vi "ParseCreators.vi"(11 "Raw HTML":string) -> (3 "Creators":T1[](array[typedef]))   [LabVIEW 2022 SP3]
uses:
  TypeDefs/Creator.ctl
  <vilib>/Utility/error.llb/Trim Whitespace One-Sided.vi
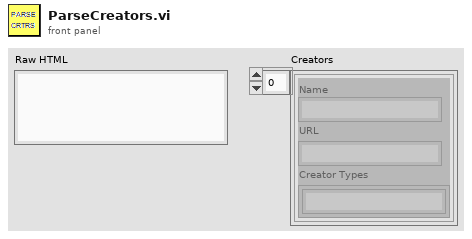
[diagram p1: front panel]
types:
  T1 = typedef "Creator.ctl" = cluster{"Name":string, "URL":string, "Creator Types":string[]}
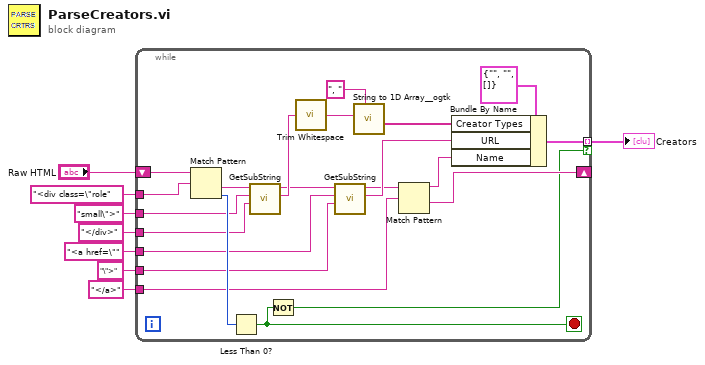
[diagram p0: block diagram]
diagram:
  n1 = while {
    shift-right: [w16] -> _
    shift-left: "Raw HTML" -> [w30]
    tunnel: "<div class=\"role" -> [w29]
    tunnel: "</div>" -> [w26]
    tunnel: "small\">" -> [w25]
    tunnel: "<a href=\"" -> [w22]
    tunnel: "\">" -> [w21]
    tunnel: "</a>" -> [w18]
    tunnel: [w15] -> w1 mode=indexing if=w13
    stop <- w14 stop-if-true
    n2 = Match Pattern(string=w30, regular expression=w29) -> (after substring=w27:string, offset past match=w28:i32)  [unwired: 1 in, 2 out]
    n3 = Less Than 0?(x=w28) -> (x < 0?=w14:bool)
    n4 = call "GetSubString.vi"("End Search"=w26, "Start Search"=w25, "String In"=w27) -> ("Match"=w24:string, "Following String Out"=w23:string)  [unwired: 6 in, 1 out]
    n5 = Not(x=w14) -> (.not. x?=w13:bool)
    n6 = call <vilib>:"Trim Whitespace.vi"("string"=w24) -> ("trimmed string"=w12:string)  [unwired: 1 in]
    n7 = call "GetSubString.vi"("End Search"=w21, "Start Search"=w22, "String In"=w23) -> ("Match"=w20:string, "Following String Out"=w19:string)  [unwired: 6 in, 1 out]
    n8 = call <userlib>:"String to 1D Array__ogtk.vi"("delimiter (Tab)"=", ", "string"=w12) -> ("Array of Strings"=w9:string[])  [unwired: 9 in]
    n9 = Match Pattern(string=w19, regular expression=w18) -> (before substring=w17:string, after substring=w16:string)  [unwired: 1 in, 2 out]
    n10 = Bundle By Name(cluster=T1 {"Name"="", "URL"="", "Creator Types"=[]} ("Creator"), "Creator Types"=w9, "URL"=w20, "Name"=w17) -> (w15:T1)
  }
  "Creators" <- w1
